vi "DCMTK_ConvertAndSend.vi"(8 "error in (no error)":errorcluster, 9 "ServerInfo":T1, 10 "Saved?":bool, 11 "File Input":string) -> (0 "error out":errorcluster, 3 "File Output":string)   [LabVIEW 2013, in "main.lvlib"]
uses:
  main.lvlib
panel:
  out "Command":string
  out "return code":i32
  out "standard error":string
  out "standard output":string
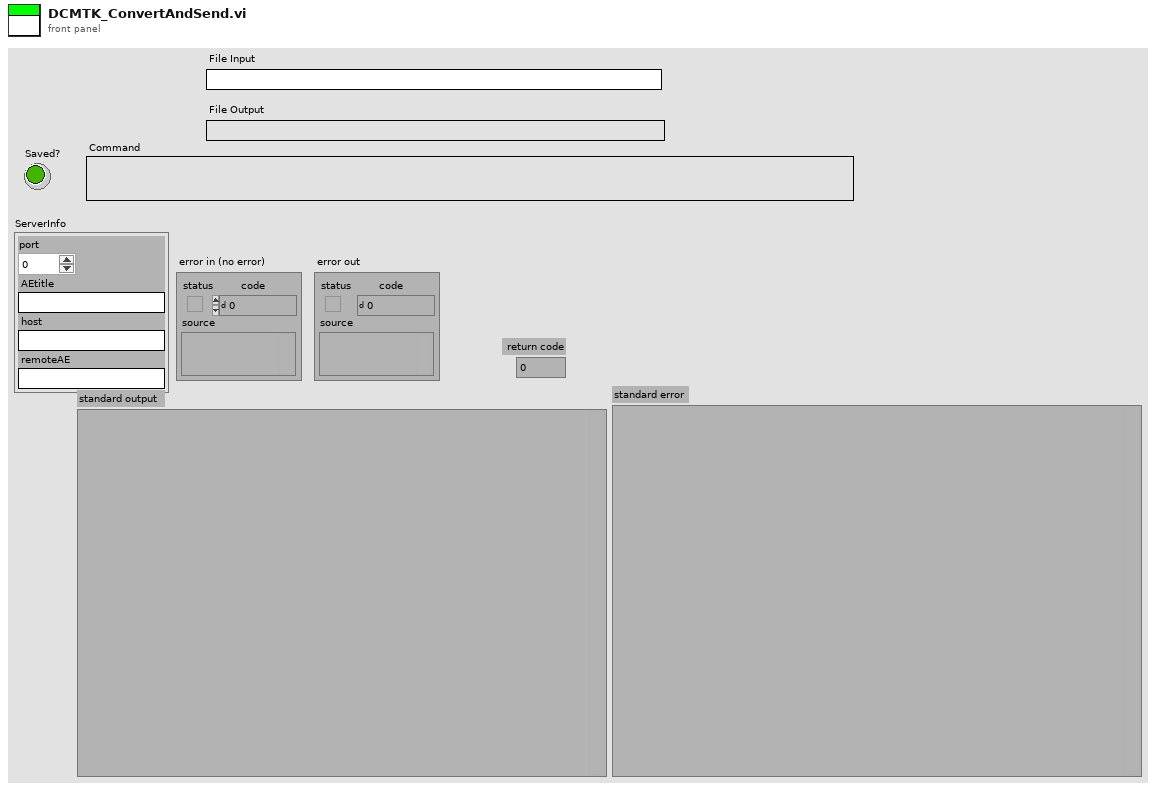
[diagram p1: front panel]
types:
  T1 = cluster{"port":i32, "AEtitle":string, "host":string, "remoteAE":string}
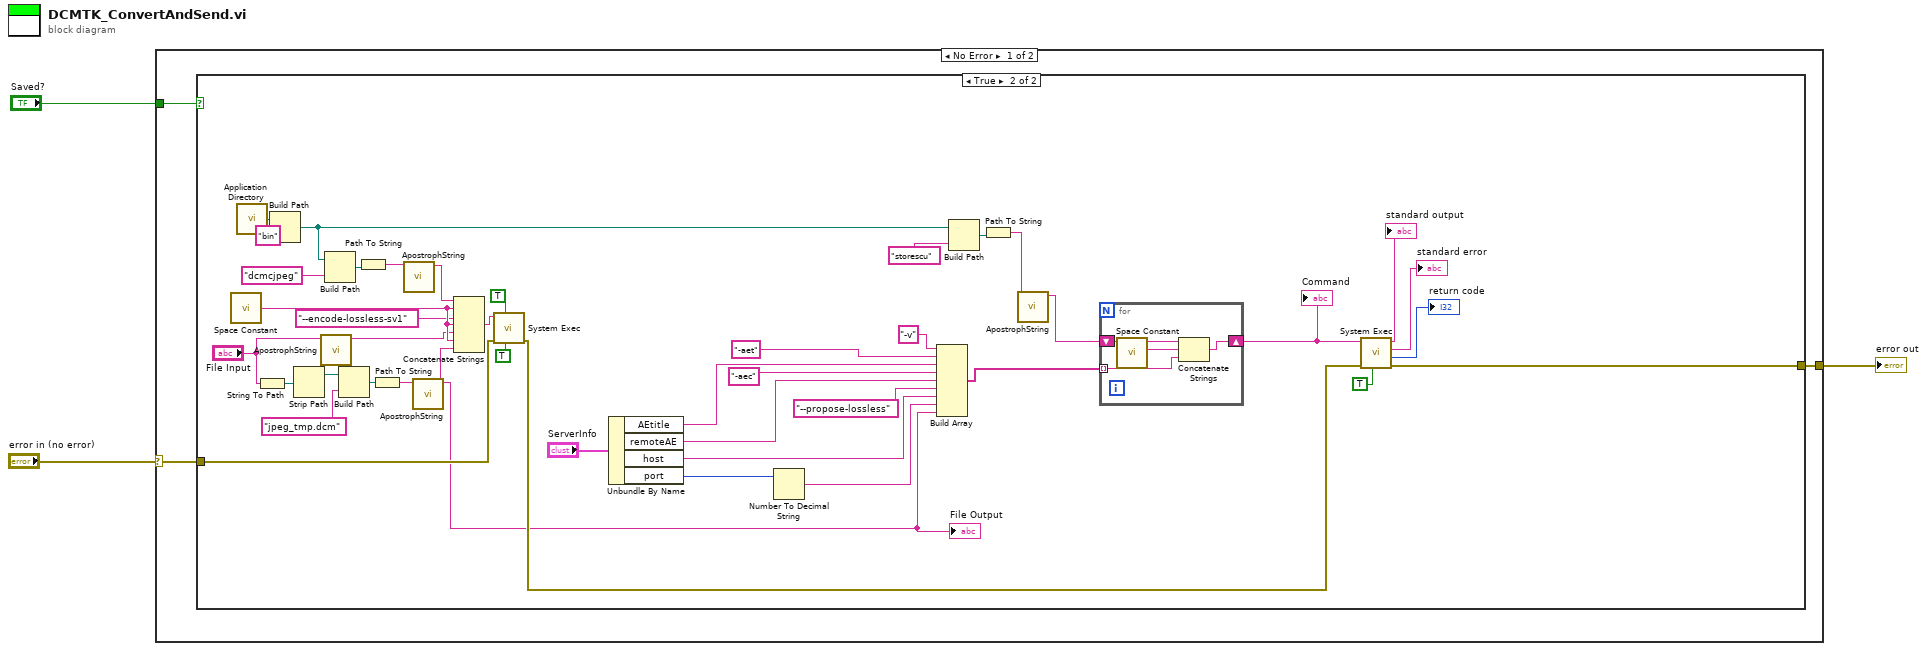
[diagram p0: block diagram]
diagram:
  n1 = case shown="No Error" "error in (no error)" {
    selector: "error in (no error)" -> [w4 w55]
    tunnel: "Saved?" -> [w6 _]
    tunnel: [w5 w55] -> w2
    frame No Error {
      n2 = case shown="True" w6 {
        tunnel: w4 -> [w7 w28]
        tunnel: [w7 w24] -> w5
        frame False {
        }
        frame True {
          n3 = call <vilib>:"Space Constant.vi"() -> ("String"=w18:string)
          n4 = call <vilib>:"Application Directory.vi"() -> ("Application Directory"=w23:path)
          n5 = String To Path(string="File Input") -> (path=w32:path)
          n6 = Build Path(base path=w23, name or relative path="bin") -> (appended path=w21:path)
          n7 = Strip Path(path=w32) -> (stripped path=w31:path)  [unwired: 1 out]
          n8 = call "ApostrophString.vi"("String in"="File Input") -> ("String out"=w12:string)  [unwired: 10 in]
          n9 = Build Path(base path=w21, name or relative path="dcmcjpeg") -> (appended path=w33:path)
          n10 = Build Path(base path=w31, name or relative path="jpeg_tmp.dcm") -> (appended path=w30:path)
          n11 = Path To String(path=w33) -> (string=w15:string)
          n12 = Path To String(path=w30) -> (string=w11:string)
          n13 = call "ApostrophString.vi"("String in"=w15) -> ("String out"=w14:string)  [unwired: 10 in]
          n14 = call "ApostrophString.vi"("String in"=w11) -> ("String out"=w10:string)  [unwired: 10 in]
          "File Output" <- w10
          n15 = Concatenate Strings(w14, w18, "--encode-lossless-sv1", w18, w12, w18, w10) -> (w16:string)
          n16 = call <vilib>:"System Exec.vi"("run minimized? (F)"=TRUE, "wait until completion? (T)"=TRUE, "error in (no error)"=w28, "command line"=w16) -> ("error out"=w27:errorcluster)  [unwired: 4 in, 3 out]
          n17 = Unbundle By Name("ServerInfo") -> ("AEtitle"=w46:string, "remoteAE"=w44:string, "host"=w42:string, "port"=w41:i32)
          n18 = Number To Decimal String(number=w41) -> (decimal integer string=w40:string)  [unwired: 1 in]
          n19 = Build Array("-v" ("element"), "-aet", w46, "-aec" ("element"), w44, "--propose-lossless" ("element"), w42, w40, w10) -> (w39:string[])
          n20 = Build Path(base path=w21, name or relative path="storescu") -> (appended path=w49:path)
          n21 = Path To String(path=w49) -> (string=w9:string)
          n22 = call "ApostrophString.vi"("String in"=w9) -> ("String out"=w8:string)  [unwired: 10 in]
          n23 = for {
            shift-right: [w53] -> w19
            shift-left: w8 -> [w54]
            tunnel: w39 -> [w52] mode=indexing
            n24 = call <vilib>:"Space Constant.vi"() -> ("String"=w51:string)
            n25 = Concatenate Strings(w54, w51, w52) -> (w53:string)
          }
          "Command" <- w19
          n26 = call <vilib>:"System Exec.vi"("run minimized? (F)"=TRUE, "error in (no error)"=w27, "command line"=w19) -> ("error out"=w24:errorcluster, "return code"=→"return code":i32, "standard error"=→"standard error":string, "standard output"=→"standard output":string)  [unwired: 5 in]
        }
      }
    }
    frame Error {
    }
  }
  "error out" <- w2
